vi "OutsideHandle_2.vi"(7 "Mode":enum16{"Open", "Read", "Write", "Close"}(ring), 8 "error in (no error)":errorcluster, 9 "data in":string, 10 "Port":u16=6342, 11 "Machine":string="localhost") -> (0 "error out":errorcluster, 1 "data out":string)   [LabVIEW 2011]
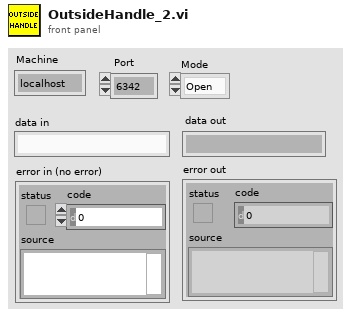
[diagram p1: front panel]
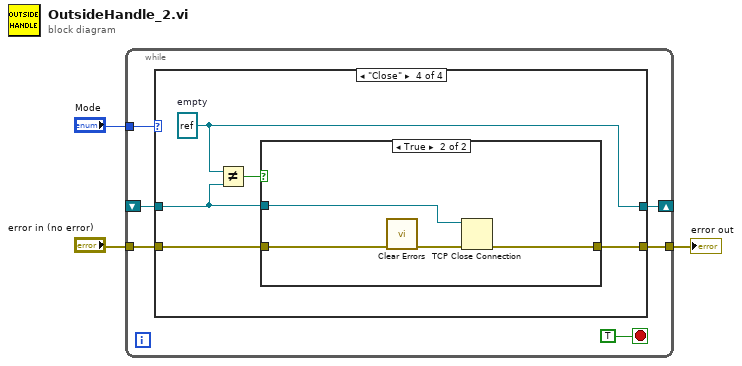
[diagram p0: block diagram]
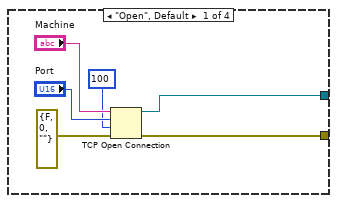
[diagram p2: hidden frame]
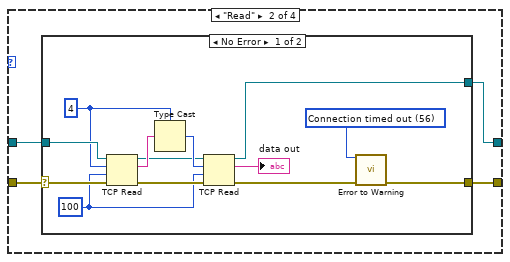
[diagram p3: hidden frame]
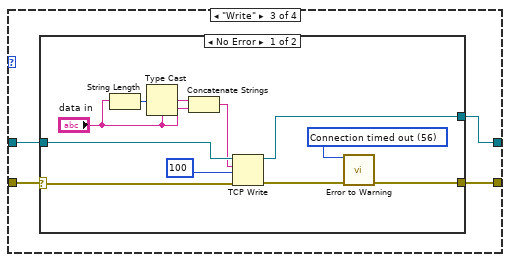
[diagram p5: hidden frame]
diagram:
  n1 = while {
    shift-right: [w9] -> _
    shift-left: _ -> [w6]
    tunnel: "Mode" -> [w5]
    tunnel: "error in (no error)" -> [w7]
    tunnel: [w8] -> w1
    stop <- TRUE stop-if-true
    n2 = case shown="\"Close\"" w5 {
      tunnel: [w12 w18 w35 w52] -> w9
      tunnel: [w10 w16 w37 w56] -> w8
      tunnel: w7 -> [_ w17 w36 w55]
      tunnel: w6 -> [_ w19 w38 w53]
      frame "Open", Default {
        n3 = TCP Open Connection(address="Machine", remote port or service name="Port", timeout ms (60000)=100, error in (no error)=errorcluster {"status"=FALSE, "code"=0, "source"=""} ("error constant")) -> (connection ID=w12:refnum<k5>, error out=w10:errorcluster)  [unwired: 1 out]
      }
      frame "Read" {
        n4 = case shown="No Error" w17 {
          selector: w17 -> [w31 w33]
          tunnel: w19 -> [w32 w34]
          tunnel: [w21 w34] -> w18
          tunnel: [w22 w33] -> w16
          frame No Error {
            w20 = 56 items=["No Error", "Argument Error", "Memory Full", "Out of Zone", "End of File", "File Already Open", "Generic File IO Error", "File Not Found", "File Permission Error", "Disk Full", "Duplicate Path", "Too Many Files Open", "Not Enabled", "Resource File Not Found", "Cannot Add Resource", "Resource Not Found", "Image Not Found", "Image Memory Error", "Pen Does Not Exist", "Config Bad Type", "Config Token Not Found", "Config Parse Error", "Config Memory Error", "Bad External Code Format", "Bad External Code Offset", "External Code Not Present", "Null Window", "Destroy Window Mixup", "Null Menu", "Print Aborted", "Bad Print Record", "Print Driver Error", "Windows Error During Print", "Memory Error During Print", "Print Dialog Error", "Generic Print Error", "Invalid Device Refnum", "Device Not Found", "Device Parameter Error", "Device Unit Error", "Can't Open Device", "Device Call Aborted", "Generic Error", "Cancelled By User", "Object ID Too Low", "Object ID Too High", "Object Not In Heap", "Unknown Heap", "Bad DefProc ID", "DefProc Not In Table", "Message Out Of Range", "Null Method", "Unknown Message", "Manager Call Not Supported", "Bad address", "Connection In progress", "Connection timed out", "Connection is already in progress", "Network attribute not supported", "Network error", "Address in use", "System out of memory", "Connection aborted", "Connection refused", "Connection is not connected", "Connection is already connected", "Connection closed", "Initialize error (interapplication manager)", "Bad occurrence", "Wait on unbound occurrence handler", "Occurrence queue overflow", "Bad path", "Semaphore not signaled", "Unrecognized type (interapplication manager)"] ("1st Error to Convert")
            w27 = 100
            w24 = 4 ("bytes to read")
            n5 = TCP Read(connection ID=w32, bytes to read=w24, error in (no error)=w31, 9:w27) -> (connection ID out=w25:refnum<k5>, data out=w26:string, error out=w28:errorcluster)  [unwired: 1 out]
            n6 = Type Cast(type=w24, x=w26) -> (*(type *) &x=w29:i32)
            n7 = TCP Read(connection ID=w25, bytes to read=w29, error in (no error)=w28, 9:w27) -> (connection ID out=w21:refnum<k5>, data out=→"data out":string, error out=w23:errorcluster)  [unwired: 1 out]
            n8 = call <vilib>:"Error to Warning.vi"("1st Error to Convert"=w20, "error in"=w23) -> ("warning out"=w22:errorcluster)  [unwired: 3 in, 10 out]
          }
          frame Error {
          }
        }
      }
      frame "Write" {
        n9 = case shown="No Error" w36 {
          selector: w36 -> [w46 w50]
          tunnel: w38 -> [w49 w51]
          tunnel: [w40 w51] -> w35
          tunnel: [w47 w50] -> w37
          frame No Error {
            w39 = 56 items=["No Error", "Argument Error", "Memory Full", "Out of Zone", "End of File", "File Already Open", "Generic File IO Error", "File Not Found", "File Permission Error", "Disk Full", "Duplicate Path", "Too Many Files Open", "Not Enabled", "Resource File Not Found", "Cannot Add Resource", "Resource Not Found", "Image Not Found", "Image Memory Error", "Pen Does Not Exist", "Config Bad Type", "Config Token Not Found", "Config Parse Error", "Config Memory Error", "Bad External Code Format", "Bad External Code Offset", "External Code Not Present", "Null Window", "Destroy Window Mixup", "Null Menu", "Print Aborted", "Bad Print Record", "Print Driver Error", "Windows Error During Print", "Memory Error During Print", "Print Dialog Error", "Generic Print Error", "Invalid Device Refnum", "Device Not Found", "Device Parameter Error", "Device Unit Error", "Can't Open Device", "Device Call Aborted", "Generic Error", "Cancelled By User", "Object ID Too Low", "Object ID Too High", "Object Not In Heap", "Unknown Heap", "Bad DefProc ID", "DefProc Not In Table", "Message Out Of Range", "Null Method", "Unknown Message", "Manager Call Not Supported", "Bad address", "Connection In progress", "Connection timed out", "Connection is already in progress", "Network attribute not supported", "Network error", "Address in use", "System out of memory", "Connection aborted", "Connection refused", "Connection is not connected", "Connection is already connected", "Connection closed", "Initialize error (interapplication manager)", "Bad occurrence", "Wait on unbound occurrence handler", "Occurrence queue overflow", "Bad path", "Semaphore not signaled", "Unrecognized type (interapplication manager)"] ("1st Error to Convert")
            n10 = String Length(string="data in") -> (length=w44:i32)
            n11 = Type Cast(type="data in", x=w44) -> (*(type *) &x=w45:string)
            n12 = Concatenate Strings(w45, "data in") -> (w42:string)
            n13 = TCP Write(connection ID=w49, data in=w42, error in (no error)=w46, 9:100 ("timeout ms (25000)")) -> (connection ID out=w40:refnum<k5>, error out=w41:errorcluster)  [unwired: 1 out]
            n14 = call <vilib>:"Error to Warning.vi"("1st Error to Convert"=w39, "error in"=w41) -> ("warning out"=w47:errorcluster)  [unwired: 3 in, 10 out]
          }
          frame Error {
          }
        }
      }
      frame "Close" {
        w52 = refnum<k5> refnum  # empty
        n15 = Not Equal?(x=w52, y=w53) -> (x != y?=w54:bool)
        n16 = case shown="True" w54 {
          tunnel: [w57 w61] -> w56
          tunnel: w55 -> [w57 w60]
          tunnel: w53 -> [_ w58]
          frame False {
          }
          frame True {
            n17 = call <vilib>:"Clear Errors.vi"("error in (no error)"=w60) -> ("error out"=w59:errorcluster)  [unwired: 6 in]
            n18 = TCP Close Connection(connection ID=w58, error in (no error)=w59) -> (error out=w61:errorcluster)  [unwired: 2 out]
          }
        }
      }
    }
  }
  "error out" <- w1
